vi "New.vi"(8 "Error In":errorcluster, 11 "Key":string) -> (0 "Error Out":errorcluster, 3 "Unescaped Variable":refnum<class "UnescapedVariable.lvclass">)   [LabVIEW 2018, in "Toolkit.lvlib" / "Tokens.lvlib" / "UnescapedVariable.lvclass"]
uses:
  UnescapedVariable.lvclass
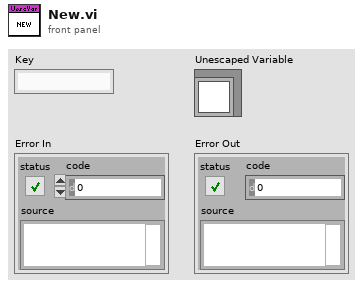
[diagram p1: front panel]
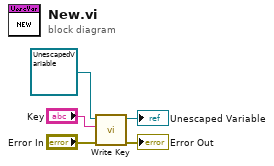
[diagram p0: block diagram]
diagram:
  n1 = call-dynamic "Write Key.vi"("Error In"="Error In", "Key"="Key", "Variable In"=refnum<class "UnescapedVariable.lvclass"> refnum ("Mustache.lvlib:Tokens.lvlib:UnescapedVariable.lvclass")) -> ("Error Out"=→"Error Out":errorcluster, "Variable Out"=→"Unescaped Variable":refnum<class "UnescapedVariable.lvclass">)  [unwired: 7 in]
